vi "Find Column Index from Property Value.vi"(7 "错误输入":cluster{"状态":bool, "代码":i32, "源":string}, 8 "通道属性值":string, 9 "通道属性名称":string, 10 "电子表格字符串数组":string[][](array[string])) -> (0 "错误输出":cluster{"状态":bool, "代码":i32, "源":string}, 2 "列索引":i32, 3 "电子表格字符串数组输出":string[][](array[string]))   [LabVIEW 2012]
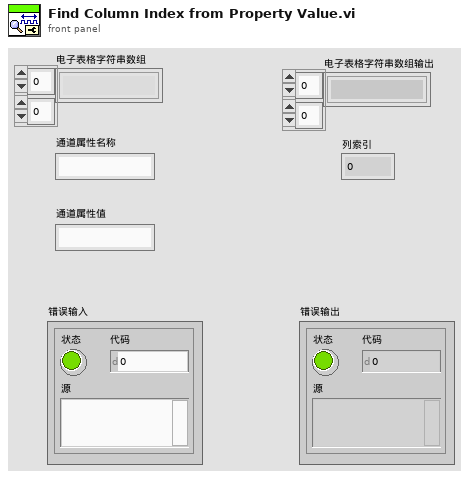
[diagram p1: front panel]
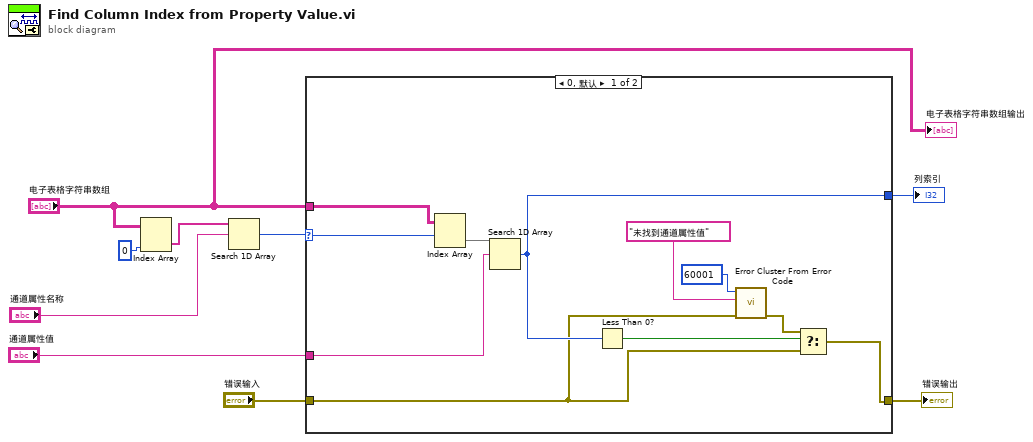
[diagram p0: block diagram]
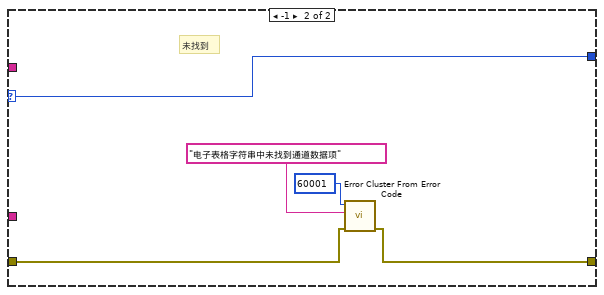
[diagram p2: hidden frame]
diagram:
  n1 = Index Array ("索引数组")(array="电子表格字符串数组", index (col)=0 ("禁用索引（列）")) -> (element=w7:string[])  [unwired: 1 in]
  n2 = Search 1D Array ("搜索一维数组")(1D array=w7, element="通道属性名称") -> (index of element=w8:i32)  [unwired: 1 in]
  n3 = case shown="0, 默认" w8 {
    selector: w8 -> [w17 w25]
    tunnel: [w16 w25] -> w9
    tunnel: "错误输入" -> [w10 w22]
    tunnel: [w11 w21] -> w4
    tunnel: "通道属性值" -> [w19 _]
    tunnel: "电子表格字符串数组" -> [w18 _]
    frame 0, Default {
      n4 = Index Array ("索引数组")(array=w18, index (row)=w17) -> (element=w20:string[])  [unwired: 1 in]
      n5 = Search 1D Array ("搜索一维数组")(1D array=w20, element=w19) -> (index of element=w16:i32)  [unwired: 1 in]
      n6 = Less Than 0? ("小于0？")(x=w16) -> (x < 0?=w15:bool)
      n7 = call <vilib>:"Error Cluster From Error Code.vi"("error in (no error)"=w10, "error message (\"\")"="未找到通道属性值" ("错误信息（“”）"), "error code (0)"=60001 ("错误代码(0)")) -> ("error out"=w12:errorcluster)  [unwired: 6 in]
      n8 = Select ("选择")(t=w12, s=w15, f=w10) -> (s? t:f=w11:cluster{"状态":bool, "代码":i32, "源":string})
    }
    frame -1 {
      # "未找到"
      n9 = call <vilib>:"Error Cluster From Error Code.vi"("error in (no error)"=w22, "error message (\"\")"="电子表格字符串中未找到通道数据项" ("错误信息（“”）"), "error code (0)"=60001 ("错误代码(0)")) -> ("error out"=w21:errorcluster)  [unwired: 6 in]
    }
  }
  "列索引" <- w9
  "错误输出" <- w4
  "电子表格字符串数组输出" <- "电子表格字符串数组"
